vi "GetConfig.vi"(6 "Enable":bool, 8 "error in (no error)":errorcluster, 10 "Cluster":T1, 11 "VISA Refnum in":refnum<visa-resource-name>) -> (0 "error out":errorcluster, 2 "output array":i32[](array[numeric]))   [LabVIEW 2020]
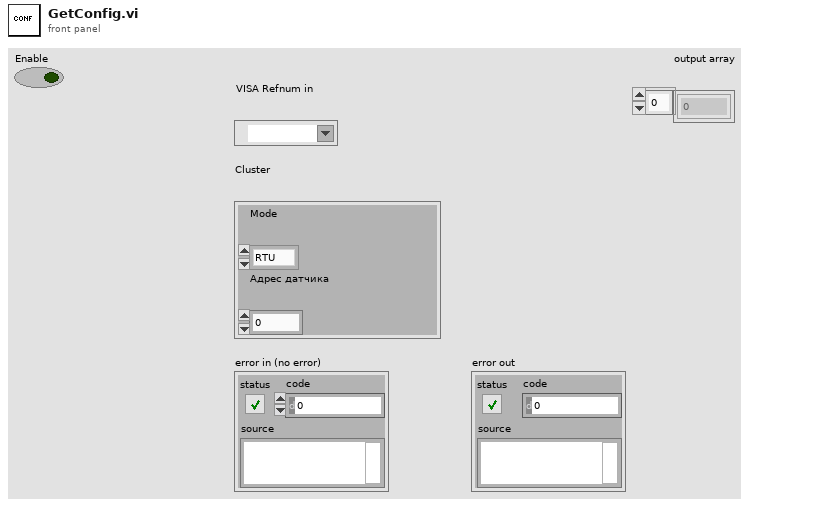
[diagram p1: front panel]
types:
  T1 = cluster{"Mode":enum16{"RTU", "ASCII"}, "Адрес датчика":u16}
  T2 = cluster{"Mode":enum16{"RTU", "ASCII"}, "Новый адрес датчика":u16}
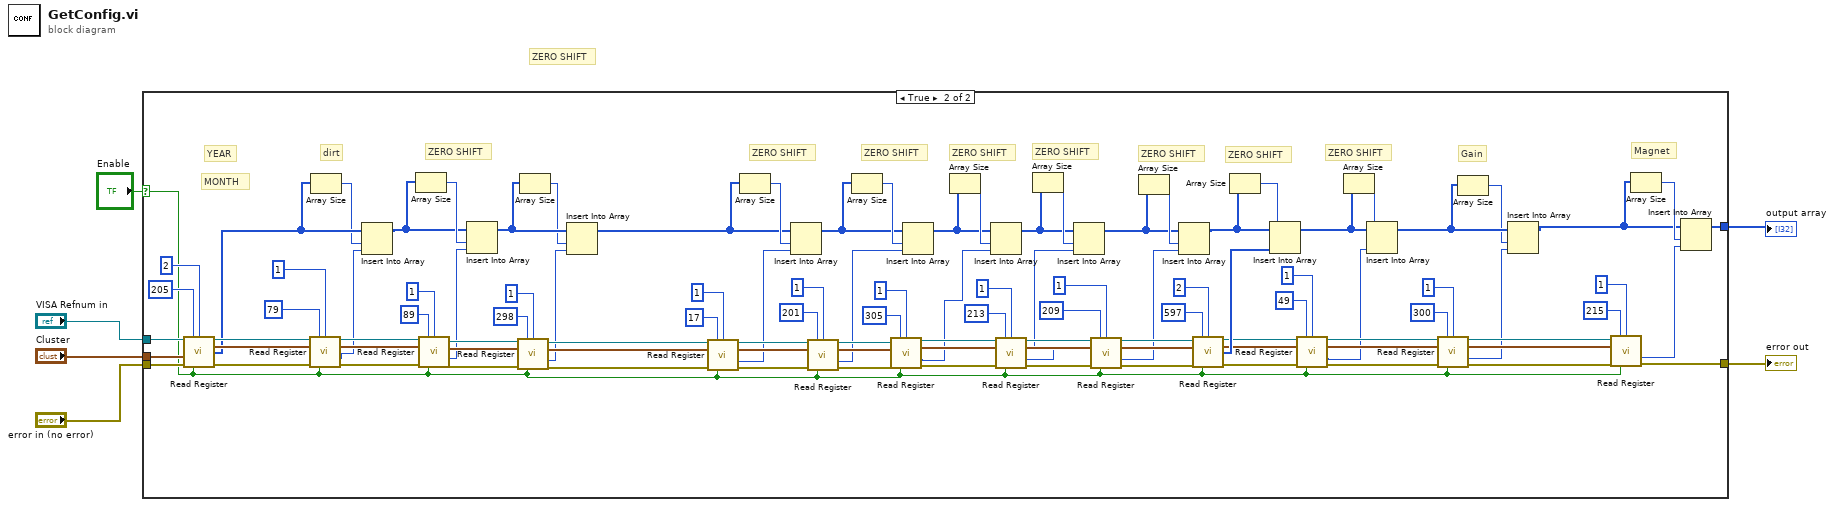
[diagram p0: block diagram]
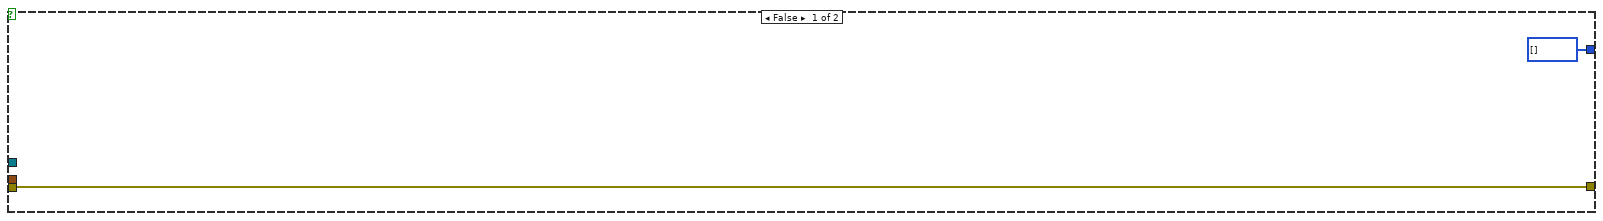
[diagram p2: hidden frame]
diagram:
  # "ZERO SHIFT"
  n1 = case shown="True" "Enable" {
    selector: "Enable" -> [_ w20]
    tunnel: "VISA Refnum in" -> [_ w110]
    tunnel: "Cluster" -> [_ w109]
    tunnel: "error in (no error)" -> [w7 w108]
    tunnel: [w7 w22] -> w3
    tunnel: [i32[] [] ("Holding Registers") w21] -> w2
    frame False {
    }
    frame True {
      # "Magnet"
      # "Gain"
      # "ZERO SHIFT"
      # "ZERO SHIFT"
      # "ZERO SHIFT"
      # "ZERO SHIFT"
      # "ZERO SHIFT"
      # "ZERO SHIFT"
      # "ZERO SHIFT"
      # "ZERO SHIFT"
      # "dirt"
      # "MONTH"
      # "YEAR"
      n2 = call "Read Register.vi"("Refnum in"=w110, "startReg"=u16 205 ("Holding Register"), "Quantity"=u16 2 ("Holding Register"), "Mode"=w109, "error in (no error)"=w108, "Enable"=w20) -> ("Refnum Out"=w105:refnum<visa-resource-name>, "ModeOut"=w104:T2, "Holding Registers"=w102:u16[], "error out"=w103:errorcluster)  [unwired: 5 in, 1 out]
      n3 = call "Read Register.vi"("Refnum in"=w105, "startReg"=u16 79 ("Holding Register"), "Quantity"=u16 1 ("Holding Register"), "Mode"=w104, "error in (no error)"=w103, "Enable"=w20) -> ("Refnum Out"=w98:refnum<visa-resource-name>, "ModeOut"=w97:T2, "Numeric"=w19:u16, "error out"=w96:errorcluster)  [unwired: 5 in, 1 out]
      n4 = Array Size(array=w102) -> (size(s)=w101:i32)
      n5 = Insert Into Array(array=w102, index=w101, new element=w19) -> (w94:u16[])
      n6 = Array Size(array=w94) -> (size(s)=w95:i32)
      n7 = call "Read Register.vi"("Refnum in"=w98, "startReg"=u16 89 ("Holding Register"), "Quantity"=u16 1 ("Holding Register"), "Mode"=w97, "error in (no error)"=w96, "Enable"=w20) -> ("Refnum Out"=w91:refnum<visa-resource-name>, "ModeOut"=w90:T2, "Numeric"=w17:u16, "error out"=w89:errorcluster)  [unwired: 5 in, 1 out]
      n8 = Insert Into Array(array=w94, index=w95, new element=w17) -> (w38:u16[])
      n9 = call "Read Register.vi"("Refnum in"=w91, "startReg"=u16 298 ("Holding Register"), "Quantity"=u16 1 ("Holding Register"), "Mode"=w90, "error in (no error)"=w89, "Enable"=w20) -> ("Refnum Out"=w86:refnum<visa-resource-name>, "ModeOut"=w85:T2, "Numeric"=w18:u16, "error out"=w84:errorcluster)  [unwired: 5 in, 1 out]
      n10 = Array Size(array=w38) -> (size(s)=w37:i32)
      n11 = Insert Into Array(array=w38, index=w37, new element=w18) -> (w39:u16[])
      n12 = call "Read Register.vi"("Refnum in"=w86, "startReg"=u16 17 ("Holding Register"), "Quantity"=u16 1 ("Holding Register"), "Mode"=w85, "error in (no error)"=w84, "Enable"=w20) -> ("Refnum Out"=w79:refnum<visa-resource-name>, "ModeOut"=w78:T2, "Numeric"=w16:u16, "error out"=w80:errorcluster)  [unwired: 5 in, 1 out]
      n13 = Array Size(array=w39) -> (size(s)=w83:i32)
      n14 = Insert Into Array(array=w39, index=w83, new element=w16) -> (w76:u16[])
      n15 = call "Read Register.vi"("Refnum in"=w79, "startReg"=u16 201 ("Holding Register"), "Quantity"=u16 1 ("Holding Register"), "Mode"=w78, "error in (no error)"=w80, "Enable"=w20) -> ("Refnum Out"=w72:refnum<visa-resource-name>, "ModeOut"=w71:T2, "Numeric"=w15:u16, "error out"=w73:errorcluster)  [unwired: 5 in, 1 out]
      n16 = Array Size(array=w76) -> (size(s)=w77:i32)
      n17 = call "Read Register.vi"("Refnum in"=w72, "startReg"=u16 305 ("Holding Register"), "Quantity"=u16 1 ("Holding Register"), "Mode"=w71, "error in (no error)"=w73, "Enable"=w20) -> ("Refnum Out"=w67:refnum<visa-resource-name>, "ModeOut"=w66:T2, "Numeric"=w14:u16, "error out"=w65:errorcluster)  [unwired: 5 in, 1 out]
      n18 = Insert Into Array(array=w76, index=w77, new element=w15) -> (w59:u16[])
      n19 = Array Size(array=w59) -> (size(s)=w70:i32)
      n20 = Insert Into Array(array=w59, index=w70, new element=w14) -> (w56:u16[])
      n21 = call "Read Register.vi"("Refnum in"=w67, "startReg"=u16 213 ("Command"), "Quantity"=u16 1, "Mode"=w66, "error in (no error)"=w65, "Enable"=w20) -> ("Refnum Out"=w62:refnum<visa-resource-name>, "ModeOut"=w61:T2, "Numeric"=w13:u16, "error out"=w60:errorcluster)  [unwired: 5 in, 1 out]
      n22 = Array Size(array=w56) -> (size(s)=w58:i32)
      n23 = Insert Into Array(array=w56, index=w58, new element=w13) -> (w55:u16[])
      n24 = call "Read Register.vi"("Refnum in"=w62, "startReg"=u16 209 ("Holding Register"), "Quantity"=u16 1 ("Holding Register"), "Mode"=w61, "error in (no error)"=w60, "Enable"=w20) -> ("Refnum Out"=w52:refnum<visa-resource-name>, "ModeOut"=w51:T2, "Numeric"=w12:u16, "error out"=w50:errorcluster)  [unwired: 5 in, 1 out]
      n25 = Array Size(array=w55) -> (size(s)=w57:i32)
      n26 = Insert Into Array(array=w55, index=w57, new element=w12) -> (w48:u16[])
      n27 = call "Read Register.vi"("Refnum in"=w52, "startReg"=u16 597 ("Command"), "Quantity"=u16 2, "Mode"=w51, "error in (no error)"=w50, "Enable"=w20) -> ("Refnum Out"=w44:refnum<visa-resource-name>, "ModeOut"=w43:T2, "Holding Registers"=w47:u16[], "error out"=w42:errorcluster)  [unwired: 5 in, 1 out]
      n28 = Array Size(array=w48) -> (size(s)=w49:i32)
      n29 = Insert Into Array(array=w48, index=w49, new element=w47) -> (w40:u16[])
      n30 = call "Read Register.vi"("Refnum in"=w44, "startReg"=u16 49 ("Holding Register"), "Quantity"=u16 1 ("Holding Register"), "Mode"=w43, "error in (no error)"=w42, "Enable"=w20) -> ("Refnum Out"=w31:refnum<visa-resource-name>, "ModeOut"=w30:T2, "Numeric"=w11:u16, "error out"=w36:errorcluster)  [unwired: 5 in, 1 out]
      n31 = Array Size(array=w40) -> (size(s)=w41:i32)
      n32 = Insert Into Array(array=w40, index=w41, new element=w11) -> (w35:u16[])
      n33 = call "Read Register.vi"("Refnum in"=w31, "startReg"=u16 300 ("Holding Register"), "Quantity"=u16 1 ("Holding Register"), "Mode"=w30, "error in (no error)"=w36, "Enable"=w20) -> ("Refnum Out"=w25:refnum<visa-resource-name>, "ModeOut"=w24:T2, "Numeric"=w10:u16, "error out"=w23:errorcluster)  [unwired: 5 in, 1 out]
      n34 = Array Size(array=w35) -> (size(s)=w34:i32)
      n35 = Insert Into Array(array=w35, index=w34, new element=w10) -> (w26:u16[])
      n36 = call "Read Register.vi"("Refnum in"=w25, "startReg"=u16 215 ("Holding Register"), "Quantity"=u16 1 ("Holding Register"), "Mode"=w24, "error in (no error)"=w23, "Enable"=w20) -> ("Numeric"=w9:u16, "error out"=w22:errorcluster)  [unwired: 5 in, 3 out]
      n37 = Array Size(array=w26) -> (size(s)=w29:i32)
      n38 = Insert Into Array(array=w26, index=w29, new element=w9) -> (w21:u16[])
    }
  }
  "error out" <- w3
  "output array" <- w2
